vi "lookup_edge_by_id.vi"(9 "destination_id":refnum<class "ID.lvclass">, 10 "source_id":refnum<class "ID.lvclass">, 11 "graph":refnum<class "DiGraph.lvclass">) -> (1 "edge":refnum<class "Edge.lvclass">, 2 "edge not found?":bool)   [LabVIEW 2020]
uses:
  ID/ID.lvclass
  edge-definition-cluster.ctl
  DiGraph.lvclass
  Edge/Edge.lvclass
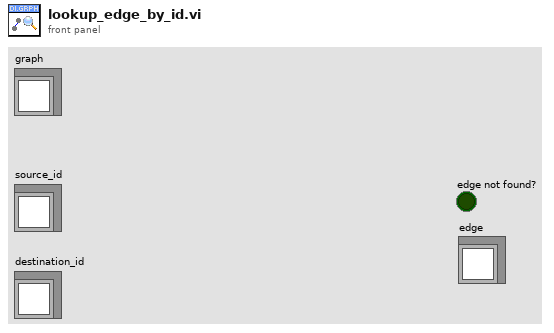
[diagram p1: front panel]
types:
  T1 = typedef "edge-definition-cluster.ctl" = cluster{"source-id":refnum<class "ID.lvclass">, "sink-id":refnum<class "ID.lvclass">}
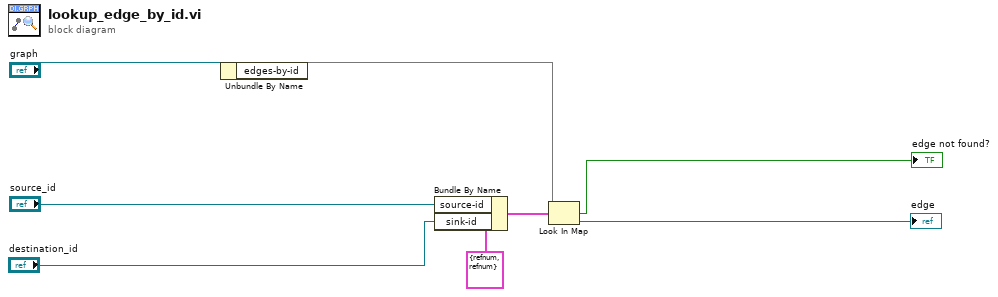
[diagram p0: block diagram]
diagram:
  n1 = Unbundle By Name("graph") -> ("edges-by-id"=w1)
  n2 = Bundle By Name(cluster=T1 {"source-id"=refnum, "sink-id"=refnum} ("nodes"), "source-id"="source_id", "sink-id"="destination_id") -> (w2:T1)
  n3 = Look In Map(map=w1, key=w2) -> (key not found?=→"edge not found?":bool, value=→"edge":refnum<class "Edge.lvclass">)  [unwired: 1 in]
